vi "Compile Engine Status.vi"(8 "error in (no error)":errorcluster, 11 "Device Item Ref in":T2 format="%.0x") -> (0 "error out":errorcluster, 2 "Status":T1, 3 "Device Item Ref out":T2 format="%.0x")   [LabVIEW 2015, in "NI 9759 RevB Custom Device.lvlib"]
uses:
  NI 9759 RevB Custom Device.lvlib
  <vilib>/NI Veristand/Custom Device API/Custom Device Item Ref.ctl
  Shared/Types/RT Status.ctl
  Shared/9759 Constants and GUIDs.vi
  <vilib>/NI VeriStand/Custom Device API/Custom Device API.lvlib
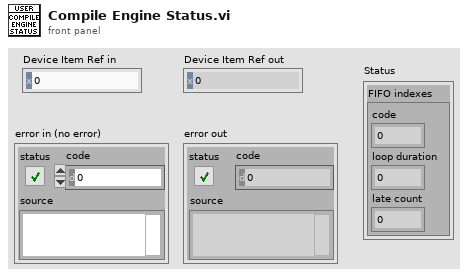
[diagram p1: front panel]
types:
  T1 = typedef "NI 9759 RevB Custom Device.lvlib/RT Status.ctl" = cluster{"FIFO indexes":cluster{"code":i32, "loop duration":i32, "late count":i32}}
  T2 = typedef "Custom Device API.lvlib/Custom Device Item Ref.ctl" = u64
  T3 = typedef "NI 9759 RevB Custom Device.lvlib/Channel.ctl" = cluster{"Name":string, "Units":string, "Default":dbl, "Description":string}
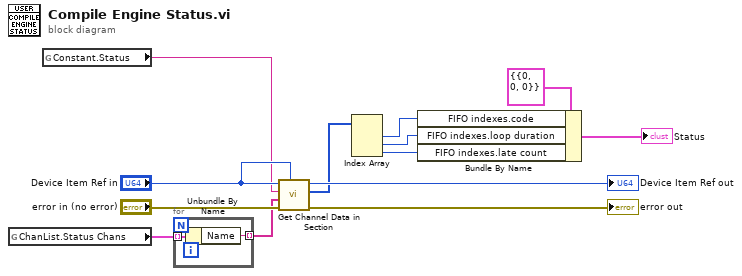
[diagram p0: block diagram]
diagram:
  n1 = global read "9759 Constants and GUIDs.vi" "ChanList.Status Chans"() -> (w1:T3[])
  n2 = global read "9759 Constants and GUIDs.vi" "Constant.Status"() -> (w2:string)
  n3 = for {
    tunnel: w1 -> [w15] mode=indexing
    tunnel: [w14] -> w9 mode=indexing
    n4 = Unbundle By Name(w15) -> ("Name"=w14:string)
  }
  n5 = call "Get Channel Data in Section.vi"("Custom device ref"="Device Item Ref in", "error in (no error)"="error in (no error)", "Channels"=w9, "Section (\"\":none)"=w2, "Item Ref in"="Device Item Ref in") -> ("error out"=→"error out":errorcluster, "FIFO indexes"=w8:i32[], "Item Ref out"=→"Device Item Ref out":T2)  [unwired: 2 in, 2 out]
  n6 = Index Array(array=w8) -> (element #1=w7:i32, element #2=w6:i32, element #3=w5:i32)  [unwired: 3 in]
  n7 = Bundle By Name(cluster=T1 {"FIFO indexes"={"code"=0, "loop duration"=0, "late count"=0}} ("Status"), "FIFO indexes.code"=w7, "FIFO indexes.loop duration"=w6, "FIFO indexes.late count"=w5) -> (→"Status":T1)
